vi "Clear_Timeout_Errors_20230511.vi"(8 "error in":errorcluster) -> (0 "error out":errorcluster)   [LabVIEW 2021]
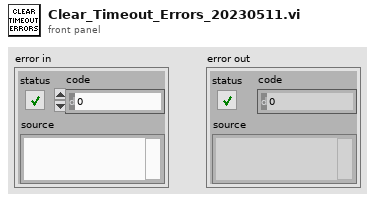
[diagram p1: front panel]
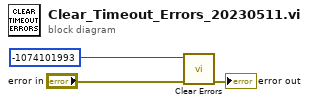
[diagram p0: block diagram]
diagram:
  n1 = call <vilib>:"Clear Errors.vi"("error in (no error)"="error in", "specific error code to clear (0: all)"=-1074101993) -> ("error out"=→"error out":errorcluster)  [unwired: 4 in, 1 out]
